vi "Buffer Data.vi"(8 "error in (no error)":errorcluster, 10 "Data":dbl, 11 "Channel Buffer DBL in":refnum<class "Channel Buffer DBL.lvclass">) -> (0 "error out":errorcluster, 3 "Channel Buffer DBL out":refnum<class "Channel Buffer DBL.lvclass">)   [LabVIEW 2020, in "VolatusHistorian.lvlib" / "Channel Buffer DBL.lvclass"]
uses:
  Channel Buffer DBL.lvclass
  Channel Buffer DBL.lvclass/Channel Buffer DBL.ctl
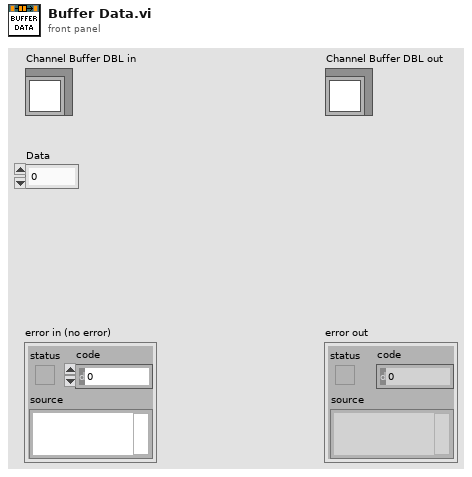
[diagram p1: front panel]
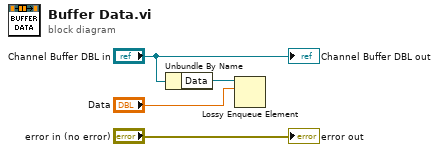
[diagram p0: block diagram]
diagram:
  n1 = Unbundle By Name("Channel Buffer DBL in") -> ("Data"=w2:refnum<queue>)
  n2 = Lossy Enqueue Element(queue=w2, element="Data") -> ()  [unwired: 1 in, 4 out]
  "error out" <- "error in (no error)"
  "Channel Buffer DBL out" <- "Channel Buffer DBL in"
